vi "GetAxisDataResults.vi"(6 "argument":i32, 7 "axisIndex":i32, 8 "error in (no error)":errorcluster, 9 "axis data signal":u32(ring) items=["AccelerationCommand"=6, "AccelerationCommandDrive"=181, "AccelerationCommandRaw"=50, "AccelerationCommandRawCal"=193, "AccelerationError"=223, "AccelerationFeedback"=192, "AccelerationMode"=144, "AccelerationRate"=140, "AccelerationTime"=138, "AccelerationType"=142, "AccuracyCorrectionEndingPosition"=418, "AccuracyCorrectionStartingPosition"=417, "AutoFocusError"=410, "AxisFault"=49, "AxisParameter"=76, "AxisStatus"=48, "Backlash"=81, "BacklashTarget"=196, "CalibrationAdjustmentState"=416, "CalibrationAdjustmentValue"=200, "CommunicationRealTimeErrors"=93, "CoordinatedDistanceRemaining"=272, "CoordinatedPositionTarget"=46, "CurrentError"=9, "CurrentFeedbackAverage"=73, "DecelerationMode"=145, "DecelerationRate"=141, "DecelerationTime"=139, "DecelerationType"=143, "DigitalInput"=15, "DigitalOutput"=16, "DistanceLog"=378, "DriveAssert"=453, "DriveCommandsDelayed"=424, "DriveCommandsLost"=425, "DriveCommunicationDelay"=253, "DriveCommunicationDelayLive"=254, "DriveInterfaceCommandCode"=191, "DriveInterfacePacketBit"=261, "DriveInterfacePacketDouble"=189, "DriveInterfacePacketFloat"=190, "DriveInterfacePacketInfoBitValue"=210, "DriveInterfacePacketInt16"=187, "DriveInterfacePacketInt32"=186, "DriveInterfacePacketInt8"=188, "DriveInterfacePacketResponseBit"=262, "DriveInterfacePacketResponseDouble"=259, "DriveInterfacePacketResponseFloat"=260, "DriveInterfacePacketResponseInt16"=257, "DriveInterfacePacketResponseInt32"=256, "DriveInterfacePacketResponseInt8"=258, "DriveInterfacePacketStreamingData"=226, "DriveMotionDelay"=199, "DriveMotionDelayLive"=252, "DriveMotionRate"=198, "DriveSMCMotionState"=168, "DriveStatus"=47, "DriveStatusActual"=99, "FeedforwardCurrent"=208, "FixtureOffset"=18, "FreezeVelocityCommand"=238, "FreezeVelocityFeedback"=239, "GainAffScale"=130, "GainKd1Scale"=333, "GainKiScale"=127, "GainKp1Scale"=334, "GainKpiScale"=129, "GainKposScale"=126, "GainKpScale"=128, "GainVffScale"=131, "GalvoLaserOffDelay"=413, "GalvoLaserOnDelay"=412, "GalvoLaserOutputRaw"=183, "GalvoLaserOutputRawAdvance"=411, "GantryMarkerLatchPosition"=368, "GantryOffset"=91, "GantryRealignState"=100, "HomeState"=82, "InternalPositionOffsets"=241, "JerkCommandRaw"=89, "JogTrajectoryStatus"=116, "MoveReferenceCornerOffset"=359, "MoveReferenceCutterOffset"=358, "MoveReferencePosition"=339, "MoveReferenceTotalOffset"=360, "NormalcyDebug"=84, "PeakCurrent"=78, "PingTest"=117, "PositionCalibration2D"=83, "PositionCalibrationAll"=55, "PositionCalibrationAllDrive"=194, "PositionCommand"=1, "PositionCommandPacket"=163, "PositionCommandRaw"=12, "PositionCommandRawBackwardsDiff"=96, "PositionCommandRawCal"=178, "PositionCommandRawUnfiltered"=227, "PositionCommandRollover"=70, "PositionError"=2, "PositionErrorGalvo"=328, "PositionFeedback"=0, "PositionFeedbackAuxiliary"=14, "PositionFeedbackAuxiliaryRollover"=71, "PositionFeedbackRollover"=69, "PositionOffset"=92, "ProgramPosition"=156, "ProgramPositionCommand"=90, "ProgramPositionFeedback"=107, "ProgramVelocityCommand"=250, "ProgramVelocityFeedback"=251, "SafeZoneState"=323, "ServoRounding"=201, "SpeedTarget"=160, "SpeedTargetActual"=266, "Stability0SettleTime"=86, "Stability1SettleTime"=87, "StatusHighLevelOffsetsLastMsec"=242, "STOStatus"=443, "SuppressedFaults"=225, "TotalMoveTime"=85, "TransformAutoOffset"=101, "TransitionOffsetErrors"=228, "VelocityCommand"=4, "VelocityCommandDrive"=180, "VelocityCommandRaw"=13, "VelocityCommandRawBackwardsDiffDelta"=97, "VelocityCommandRawCal"=179, "VelocityError"=5, "VelocityFeedback"=3, "VelocityFeedbackAverage"=72], 10 "Data In":refnum<k24>, 11 "controller in":refnum<k24>) -> (0 "error out":errorcluster, 1 "AxisData":dbl[](array[numeric]), 2 "Data Out":refnum<k24>, 3 "controller out":refnum<k24>)   [LabVIEW 2010]
uses:
  c:/aerotech/controller/stable/a3200/pc/labview/2010/bin/Aerotech.A3200.dll
  bin/Aerotech.A3200.dll
  c:/aerotech/controller/stable/a3200/pc/labview/2010/bin/Aerotech.A3200.LabVIEW.dll
  bin/Aerotech.A3200.LabVIEW.dll
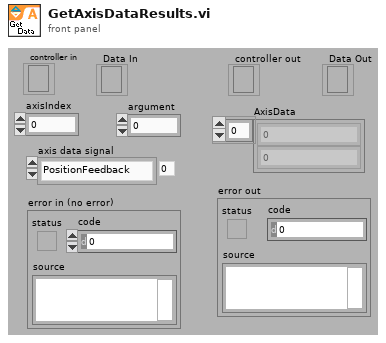
[diagram p1: front panel]
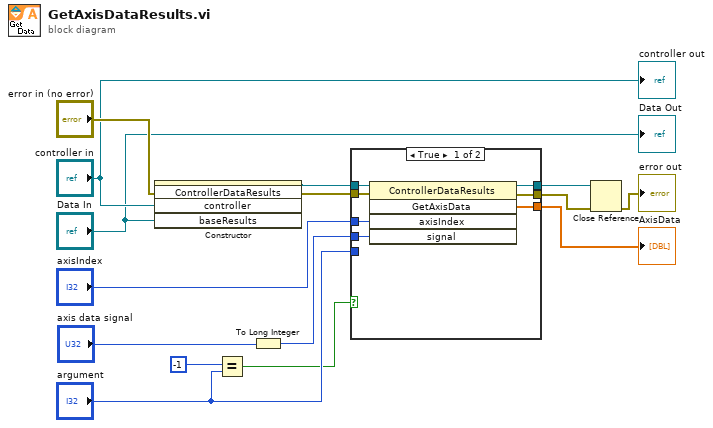
[diagram p0: block diagram]
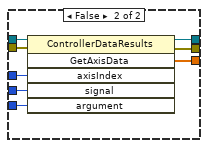
[diagram p2: hidden frame]
diagram:
  n1 = constructor class="ControllerDataResults"(error in="error in (no error)", "controller"="controller in", "baseResults"="Data In") -> (reference out=w14:refnum<k24>, error out=w13:errorcluster)  [unwired: 2 in, 3 out]
  n2 = Equal?(x=-1, y="argument") -> (x = y?=w5:bool)
  n3 = To Long Integer(number="axis data signal") -> (32bit integer=w4:i32)
  n4 = case shown="True" w5 {
    tunnel: "axisIndex" -> [w22 w30]
    tunnel: [w21 w29] -> w3
    tunnel: [w20 w28] -> w2
    tunnel: w14 -> [w19 w27]
    tunnel: w13 -> [w18 w26]
    tunnel: w4 -> [w17 w25]
    tunnel: "argument" -> [_ w23]
    tunnel: [w16 w24] -> w12
    frame True {
      n5 = invoke class="ControllerDataResults" method="GetAxisData"(reference=w19, error in=w18, "axisIndex"=w22, "signal"=w17) -> (reference out=w20:refnum<k24>, error out=w21:errorcluster, "GetAxisData"=w16:dbl[])  [unwired: 1 in, 2 out]
    }
    frame False {
      n6 = invoke class="ControllerDataResults" method="GetAxisData"(reference=w27, error in=w26, "axisIndex"=w30, "signal"=w25, "argument"=w23) -> (reference out=w28:refnum<k24>, error out=w29:errorcluster, "GetAxisData"=w24:dbl[])  [unwired: 1 in, 3 out]
    }
  }
  "AxisData" <- w12
  n7 = Close Reference(reference=w2, error in (no error)=w3) -> (error out=→"error out":errorcluster)
  "controller out" <- "controller in"
  "Data Out" <- "Data In"
